vi "CRYGet Curve Library Arr.vi"(9 "Index":i32[](array[numeric]), 10 "sOption":string, 11 "Type In":enum16{"Curves", "Values", "Results", "WFM"}(ring)) -> (1 "Waveforms":T1 {"Y dB ref" format="%.1f"; "Y axis" items=["Log", "Lin"]; "Y data" items=["dB", "Lin"]; "X data" items=["dB", "Lin"]}, 2 "Results":T3 {"Margin" format="%.2f"}, 3 "Curves/Values":T5 {"Z data" items=["dB", "Lin"]; "X data" items=["dB", "Lin"]; "Y data" items=["dB", "Lin"]; "Z dB ref" format="%.1f"; "Z axis" items=["Log", "Lin"]; "X dB ref" format="%.1f"; "X axis" items=["Log", "Lin"]; "Y axis" items=["Log", "Lin"]; "Y dB ref" format="%.1f"; "Curve"."z" format="%.2f"; "Curve"."y" format="%.2f"; "Curve"."x" format="%.2f"})   [LabVIEW 2013]
uses:
  CRYSystem/Typedef Control/CRYData Cluster Array.ctl
  CRYSystem/Typedef Control/CRYData Cluster.ctl
  CRYSystem/Typedef Control/CRYResult Cluster Array.ctl
  CRYSystem/Typedef Control/CRYResult Cluster.ctl
  CRYSystem/Typedef Control/CRYWaveform Cluster Array.ctl
  CRYSystem/Typedef Control/CRYWaveform Cluster.ctl
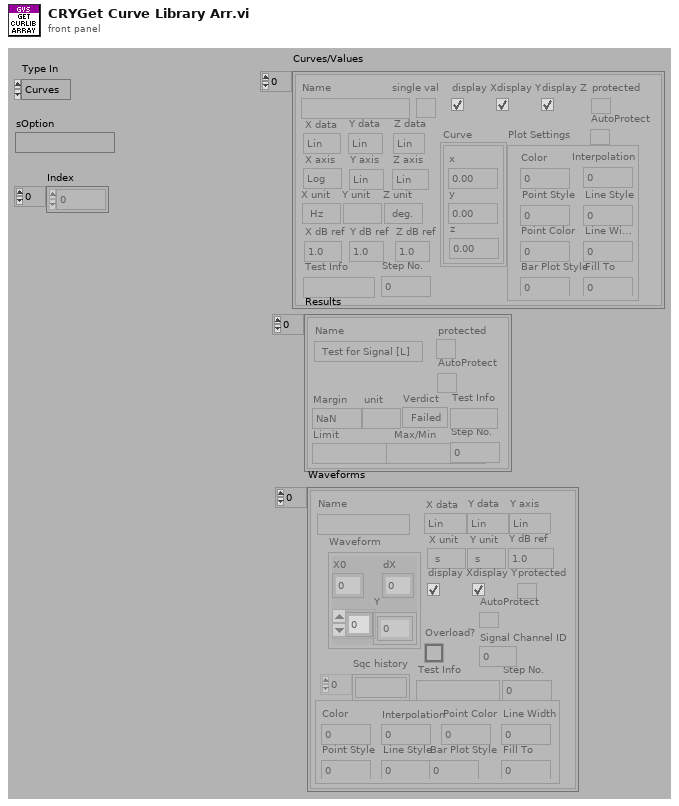
[diagram p1: front panel]
types:
  T1 = typedef "CRYWaveform Cluster Array.ctl" = T2[]
  T2 = typedef "CRYWaveform Cluster.ctl" = cluster{"Waveform":cluster{"X0":dbl, "dX":dbl, "Y":sgl[]}, "X data":u16, "Y data":u16, "Y axis":u16, "X unit":string, "Y unit":string, "Y dB ref":dbl, "display Y":bool, "display X":bool, "Overload?":bool, "Test Info":string, "Step No.":i32, "Name":string, "protected":bool, "Sqc history":string[], "Signal Channel ID":i32, "Plot Settings":cluster{"Color":u32, "Interpolation":u8, "Point Style":u8, "Line Style":u8, "Point Color":u32, "Line Width":u8, "Bar Plot Style":u8, "Fill To":i16}, "AutoProtect":bool}
  T3 = typedef "CRYResult Cluster Array.ctl" = T4[]
  T4 = typedef "CRYResult Cluster.ctl" = cluster{"Name":string, "Margin":dbl, "unit":string, "Verdict":bool, "Limit":string, "Max/Min":string, "protected":bool, "Step No.":i32, "Test Info":string, "AutoProtect":bool}
  T5 = typedef "CRYData Cluster Array.ctl" = T6[]
  T6 = typedef "CRYData Cluster.ctl" = cluster{"Name":string, "Curve":cluster{"x":dbl, "y":dbl, "z":dbl}[], "X data":u16, "Y data":u16, "Z data":u16, "X axis":u16, "Y axis":u16, "Z axis":u16, "X unit":string, "Y unit":string, "Z unit":string, "X dB ref":dbl, "Y dB ref":dbl, "Z dB ref":dbl, "single val":bool, "protected":bool, "display X":bool, "display Y":bool, "display Z":bool, "Test Info":string, "Step No.":i32, "Plot Settings":cluster{"Color":u32, "Interpolation":u8, "Point Style":u8, "Line Style":u8, "Point Color":u32, "Line Width":u8, "Bar Plot Style":u8, "Fill To":i16}, "AutoProtect":bool}
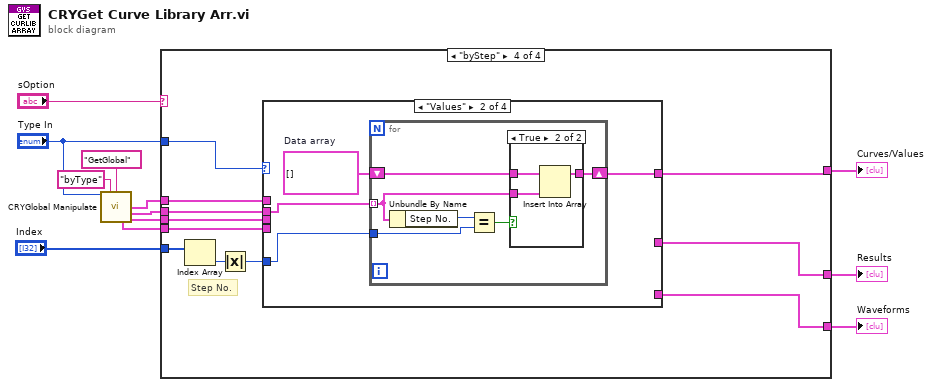
[diagram p0: block diagram]
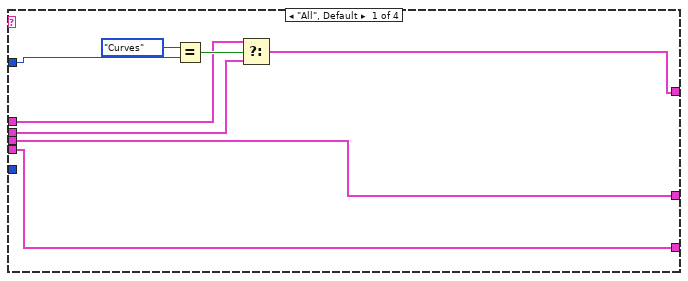
[diagram p2: hidden frame]
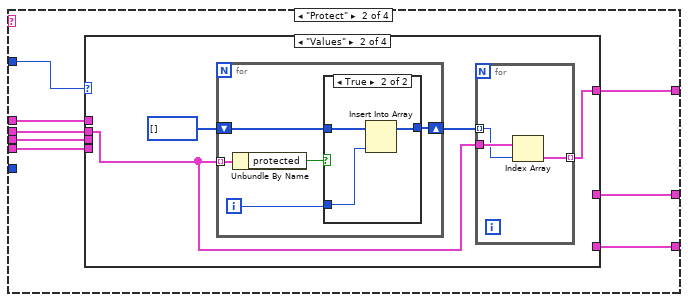
[diagram p3: hidden frame]
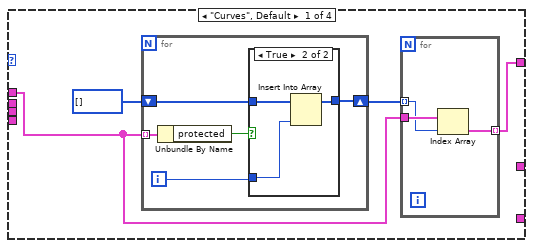
[diagram p4: hidden frame]
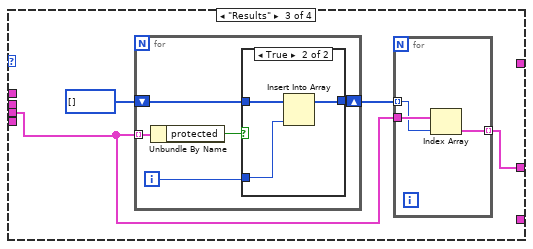
[diagram p7: hidden frame]
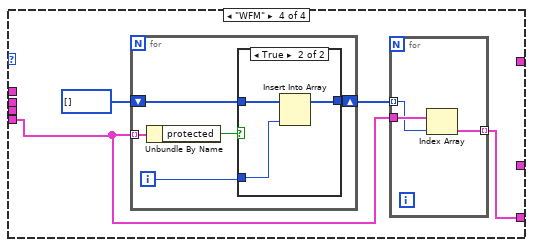
[diagram p9: hidden frame]
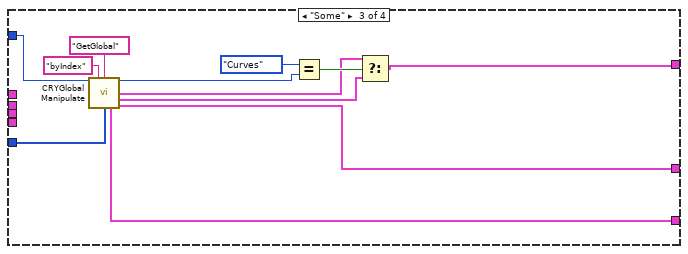
[diagram p11: hidden frame]
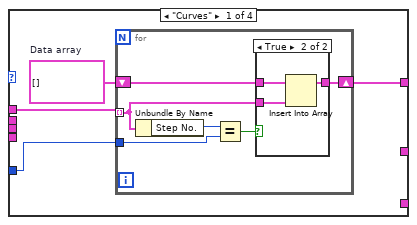
[diagram p12: hidden frame]
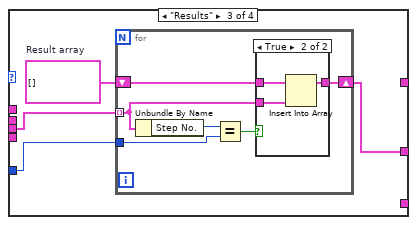
[diagram p15: hidden frame]
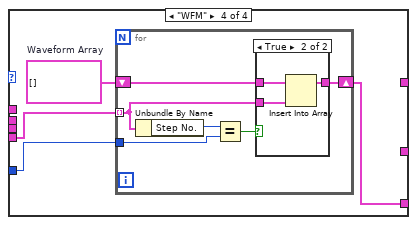
[diagram p17: hidden frame]
diagram:
  n1 = call "CRYGlobal Manipulate.vi"("Type"="Type In", "sOption"="byType", "sAction"="GetGlobal") -> ("Curves Out"=w3:T6[], "Values Out"=w6:T6[], "WFM Out"=w4:T2[], "Results Out"=w5:T4[])  [unwired: 6 in, 3 out]
  n2 = case shown="\"byStep\"" "sOption" {
    tunnel: [w13 w28 w95 w113] -> w12
    tunnel: [w20 w27 w94 w111] -> w11
    tunnel: [w19 w26 w93 w112] -> w10
    tunnel: "Index" -> [_ _ w102 w114]
    tunnel: w6 -> [w15 w25 _ w109]
    tunnel: w5 -> [w20 w24 _ w108]
    tunnel: w4 -> [w19 w22 _ w107]
    tunnel: "Type In" -> [w17 w23 w101 w110]
    tunnel: w3 -> [w14 w21 _ w106]
    frame "All", Default {
      n3 = Equal?(x=enum16{"Curves", "Values", "Results", "WFM"}."Curves", y=w17) -> (x = y?=w18:bool)
      n4 = Select(t=w14, s=w18, f=w15) -> (s? t:f=w13:T6[])
    }
    frame "Protect" {
      n5 = case shown="\"Values\"" w23 {
        tunnel: [w30 w46 _ _] -> w28
        tunnel: [_ _ w62 _] -> w27
        tunnel: [_ _ _ w78] -> w26
        tunnel: w25 -> [_ w45 _ _]
        tunnel: w24 -> [_ _ w61 _]
        tunnel: w22 -> [_ _ _ w77]
        tunnel: w21 -> [w29 _ _ _]
        frame "Curves", Default {
          n6 = for {
            tunnel: w29 -> [w40] mode=indexing
            shift-right: [w38] -> w31
            shift-left: i32[] [] -> [w39]
            i -> [w37]
            n7 = Unbundle By Name(w40) -> ("protected"=w36:bool)
            n8 = case shown="True" w36 {
              tunnel: [w41 w43] -> w38
              tunnel: w39 -> [w41 w44]
              tunnel: w37 -> [_ w42]
              frame False {
              }
              frame True {
                n9 = Insert Into Array(array=w44, new element=w42) -> (w43:i32[])  [unwired: 1 in]
              }
            }
          }
          n10 = for {
            tunnel: w31 -> [w34] mode=indexing
            tunnel: w29 -> [w35]
            tunnel: [w33] -> w30 mode=indexing
            n11 = Index Array(array=w35, index=w34) -> (element=w33:T6)
          }
        }
        frame "Values" {
          n12 = for {
            tunnel: w45 -> [w56] mode=indexing
            shift-right: [w54] -> w47
            shift-left: i32[] [] -> [w55]
            i -> [w53]
            n13 = Unbundle By Name(w56) -> ("protected"=w52:bool)
            n14 = case shown="True" w52 {
              tunnel: [w57 w59] -> w54
              tunnel: w55 -> [w57 w60]
              tunnel: w53 -> [_ w58]
              frame False {
              }
              frame True {
                n15 = Insert Into Array(array=w60, new element=w58) -> (w59:i32[])  [unwired: 1 in]
              }
            }
          }
          n16 = for {
            tunnel: w47 -> [w50] mode=indexing
            tunnel: w45 -> [w51]
            tunnel: [w49] -> w46 mode=indexing
            n17 = Index Array(array=w51, index=w50) -> (element=w49:T6)
          }
        }
        frame "Results" {
          n18 = for {
            tunnel: w61 -> [w72] mode=indexing
            shift-right: [w70] -> w63
            shift-left: i32[] [] -> [w71]
            i -> [w69]
            n19 = Unbundle By Name(w72) -> ("protected"=w68:bool)
            n20 = case shown="True" w68 {
              tunnel: [w73 w75] -> w70
              tunnel: w71 -> [w73 w76]
              tunnel: w69 -> [_ w74]
              frame False {
              }
              frame True {
                n21 = Insert Into Array(array=w76, new element=w74) -> (w75:i32[])  [unwired: 1 in]
              }
            }
          }
          n22 = for {
            tunnel: w63 -> [w66] mode=indexing
            tunnel: w61 -> [w67]
            tunnel: [w65] -> w62 mode=indexing
            n23 = Index Array(array=w67, index=w66) -> (element=w65:T4)
          }
        }
        frame "WFM" {
          n24 = for {
            tunnel: w77 -> [w88] mode=indexing
            shift-right: [w86] -> w79
            shift-left: i32[] [] -> [w87]
            i -> [w85]
            n25 = Unbundle By Name(w88) -> ("protected"=w84:bool)
            n26 = case shown="True" w84 {
              tunnel: [w89 w91] -> w86
              tunnel: w87 -> [w89 w92]
              tunnel: w85 -> [_ w90]
              frame False {
              }
              frame True {
                n27 = Insert Into Array(array=w92, new element=w90) -> (w91:i32[])  [unwired: 1 in]
              }
            }
          }
          n28 = for {
            tunnel: w79 -> [w82] mode=indexing
            tunnel: w77 -> [w83]
            tunnel: [w81] -> w78 mode=indexing
            n29 = Index Array(array=w83, index=w82) -> (element=w81:T2)
          }
        }
      }
    }
    frame "Some" {
      n30 = call "CRYGlobal Manipulate.vi"("Type"=w101, "sOption"="byIndex", "sAction"="GetGlobal", "nData"=w102) -> ("Type out"=w98:enum16{"Curves", "Values", "Results", "WFM"}, "Curves Out"=w97:T6[], "Values Out"=w96:T6[], "WFM Out"=w93:T2[], "Results Out"=w94:T4[])  [unwired: 5 in, 2 out]
      n31 = Equal?(x=enum16{"Curves", "Values", "Results", "WFM"}."Curves", y=w98) -> (x = y?=w100:bool)
      n32 = Select(t=w97, s=w100, f=w96) -> (s? t:f=w95:T6[])
    }
    frame "byStep" {
      # "Step No."
      n33 = Index Array(array=w114) -> (element=w115:i32)  [unwired: 1 in]
      n34 = Absolute Value(x=w115) -> (abs(x)=w105:i32)
      n35 = case shown="\"Values\"" w110 {
        tunnel: w108 -> [_ _ w146 _]
        tunnel: w107 -> [_ _ _ w158]
        tunnel: w105 -> [w119 w133 w147 w161]
        tunnel: [w118 w132 _ _] -> w113
        tunnel: w109 -> [_ w130 _ _]
        tunnel: [_ _ _ w159] -> w112
        tunnel: [_ _ w144 _] -> w111
        tunnel: w106 -> [w116 _ _ _]
        frame "Curves" {
          w117 = T5 []  # Data array
          n36 = for {
            tunnel: w116 -> [w120] mode=indexing
            tunnel: w119 -> [w124]
            shift-right: [w122] -> w118
            shift-left: w117 -> [w121]
            n37 = Unbundle By Name(w120) -> ("Step No."=w125:i32)
            n38 = Equal?(x=w125, y=w124) -> (x = y?=w123:bool)
            n39 = case shown="True" w123 {
              tunnel: [w126 w128] -> w122
              tunnel: w121 -> [w126 w129]
              tunnel: w120 -> [_ w127]
              frame False {
              }
              frame True {
                n40 = Insert Into Array(array=w129, new element=w127) -> (w128:T5)  [unwired: 1 in]
              }
            }
          }
        }
        frame "Values" {
          w131 = T5 []  # Data array
          n41 = for {
            tunnel: w130 -> [w134] mode=indexing
            tunnel: w133 -> [w138]
            shift-right: [w136] -> w132
            shift-left: w131 -> [w135]
            n42 = Unbundle By Name(w134) -> ("Step No."=w139:i32)
            n43 = Equal?(x=w139, y=w138) -> (x = y?=w137:bool)
            n44 = case shown="True" w137 {
              tunnel: [w140 w142] -> w136
              tunnel: w135 -> [w140 w143]
              tunnel: w134 -> [_ w141]
              frame False {
              }
              frame True {
                n45 = Insert Into Array(array=w143, new element=w141) -> (w142:T5)  [unwired: 1 in]
              }
            }
          }
        }
        frame "Results" {
          w145 = T3 []  # Result array
          n46 = for {
            tunnel: w146 -> [w148] mode=indexing
            tunnel: w147 -> [w152]
            shift-right: [w150] -> w144
            shift-left: w145 -> [w149]
            n47 = Unbundle By Name(w148) -> ("Step No."=w153:i32)
            n48 = Equal?(x=w153, y=w152) -> (x = y?=w151:bool)
            n49 = case shown="True" w151 {
              tunnel: [w154 w156] -> w150
              tunnel: w149 -> [w154 w157]
              tunnel: w148 -> [_ w155]
              frame False {
              }
              frame True {
                n50 = Insert Into Array(array=w157, new element=w155) -> (w156:T3)  [unwired: 1 in]
              }
            }
          }
        }
        frame "WFM" {
          w160 = T1 []  # Waveform Array
          n51 = for {
            tunnel: w158 -> [w162] mode=indexing
            tunnel: w161 -> [w166]
            shift-right: [w164] -> w159
            shift-left: w160 -> [w163]
            n52 = Unbundle By Name(w162) -> ("Step No."=w167:i32)
            n53 = Equal?(x=w167, y=w166) -> (x = y?=w165:bool)
            n54 = case shown="True" w165 {
              tunnel: [w168 w170] -> w164
              tunnel: w163 -> [w168 w171]
              tunnel: w162 -> [_ w169]
              frame False {
              }
              frame True {
                n55 = Insert Into Array(array=w171, new element=w169) -> (w170:T1)  [unwired: 1 in]
              }
            }
          }
        }
      }
    }
  }
  "Curves/Values" <- w12
  "Results" <- w11
  "Waveforms" <- w10
